vi "Read Inbound Message.vi"(8 "error in (no error)":errorcluster, 11 "MQTT Server":refnum<class "Server.lvclass">) -> (0 "error out":errorcluster, 2 "Inbound Message":refnum<user-event>, 3 "MQTT Server":refnum<class "Server.lvclass">)   [LabVIEW 2013, in "MQTT Server.lvlib" / "Server.lvclass"]
uses:
  Server.lvclass
  <vilib>/LabVIEW Open Source Project/MQTT Control Packets/Control Packets/PUBLISH/PUBLISH.lvclass
  <vilib>/LabVIEW Open Source Project/MQTT Connection/MQTT_Base/Base Class/MQTT_Base.lvclass/MQTT_Base.ctl
  <vilib>/LabVIEW Open Source Project/MQTT Connection/MQTT_Base/Base Class/MQTT_Base.lvclass
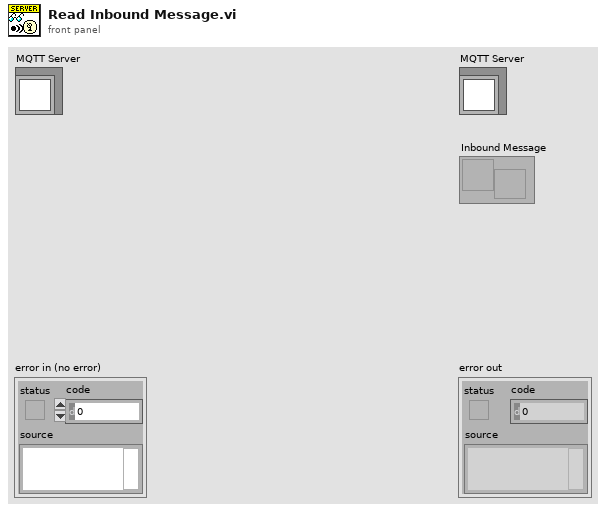
[diagram p1: front panel]
types:
  T1 = typedef "MQTT Base.lvlib/MQTT_Base.lvclass/Public Events -- cluster.ctl" = cluster{"Stop Event":refnum<user-event>, "Error Event":refnum<user-event>, "Inbound Message":refnum<user-event>}
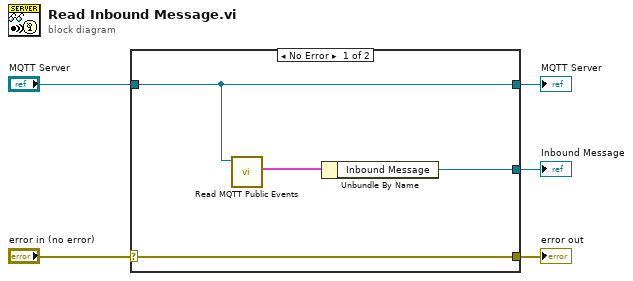
[diagram p0: block diagram]
diagram:
  n1 = case shown="No Error" "error in (no error)" {
    selector: "error in (no error)" -> [w9 w10]
    tunnel: [w9 w10] -> w4
    tunnel: [w8 w11] -> w2
    tunnel: "MQTT Server" -> [w8 w11]
    tunnel: [w6 _] -> w1
    frame No Error {
      n2 = call <vilib>:"Read MQTT Public Events.vi"("MQTT_Base in"=w8) -> ("MQTT Public Events"=w7:T1)  [unwired: 8 in, 2 out]
      n3 = Unbundle By Name(w7) -> ("Inbound Message"=w6:refnum<user-event>)
    }
    frame Error {
    }
  }
  "error out" <- w4
  "MQTT Server" <- w2
  "Inbound Message" <- w1
